vi "Stream to AVI Files (Optimized Performance) ajg.vi"() -> ()   [LabVIEW 2020]
doc: "The Stream to AVI Files (Optimized Performance) example shows how to save images to an AVI file when using a ring acquisition. This example uses a ring acquisition which is optimized for performance, but has some restrictions on the camera's image format and size. Use the Stream to AVI File example if your camera settings do not work with a ring acquisition."
uses:
  <vilib>/vision/Avi.llb/IMAQ AVI2 Codec Path.ctl
  <vilib>/vision/driver/IMAQdx.llb/IMAQdx Acquisition Mode.ctl
  <vilib>/vision/Image Controls.llb/IMAQ Image.ctl
  <vilib>/vision/driver/IMAQdx.llb/IMAQdx Buffer Number Mode.ctl
  <vilib>/Utility/High Resolution Relative Seconds.vi
  <vilib>/vision/driver/NI_Vision_Acquisition_Software.lvlib
  <resource>/objmgr/imaqdx.rc
panel:
  in  "Destination Folder":path
  in  "Skip Count":u32
  out "Images Saved Per Second":dbl
  out "Images Acquired Per Second":dbl
  in  "Images per AVI":i32=100
  out "Write Speed":dbl(graph) caption="Image File Write Speed"
  in  "Start":bool
  in  "Codec":u16(ring) items=["FF Video Codec 1 (FFV1) (NI Vision)", "Motion JPEG (NI Vision)", "VP8 (NI Vision)", "VP9 (NI Vision)", "Y800 Uncompressed Grey Scale (NI Vision)", "YUV 4:2:0 Planar (NI Vision)"]
  out "Images Behind":i32
  in  "Number of Images":i32=30
  in  "Camera Name":refnum<k21> caption="IMAQdx Session"
  in  "Stop":bool
  # "Overview: Demonstrates how to stream images to an AVI file when using a ring acquisition.\nRequirements: Vision Acquisition Software\nInstructions:\n1. Select the Camera Name\n2. Run the VI\n3. Select the Codec and click Start.\n4. Increase the Skip Count if Images Behind is greater than 0."
  # "Use the skip count to skip acquiring some images so the image logging can avoid getting behind."
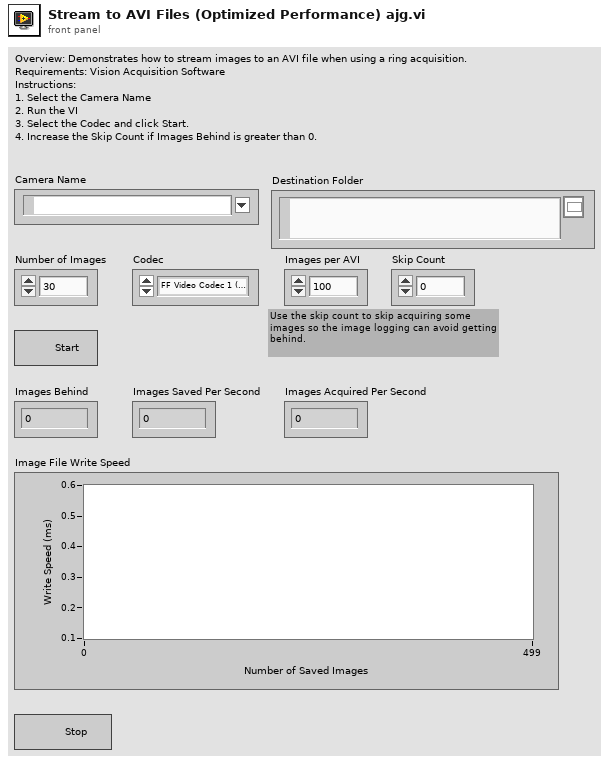
[diagram p1: front panel]
types:
  T1 = typedef "IMAQ AVI2 Codec Path.ctl" = u32
  T2 = typedef "IMAQdx.ctl" = refnum<k21>
  T3 = typedef "IMAQ Image.ctl" = refnum<image>
  T4 = typedef "NI_Vision_Acquisition_Software.lvlib/IMAQdx Acquisition Mode.ctl" = enum32{"One Shot", "Continuous"}
  T5 = typedef "NI_Vision_Acquisition_Software.lvlib/IMAQdx Buffer Number Mode.ctl" = enum32{"Next", "Last", "Buffer Number", "Every", "Last New"}
  T6 = typedef "IMAQ AVI2 Refnum.ctl" = refnum<k20>
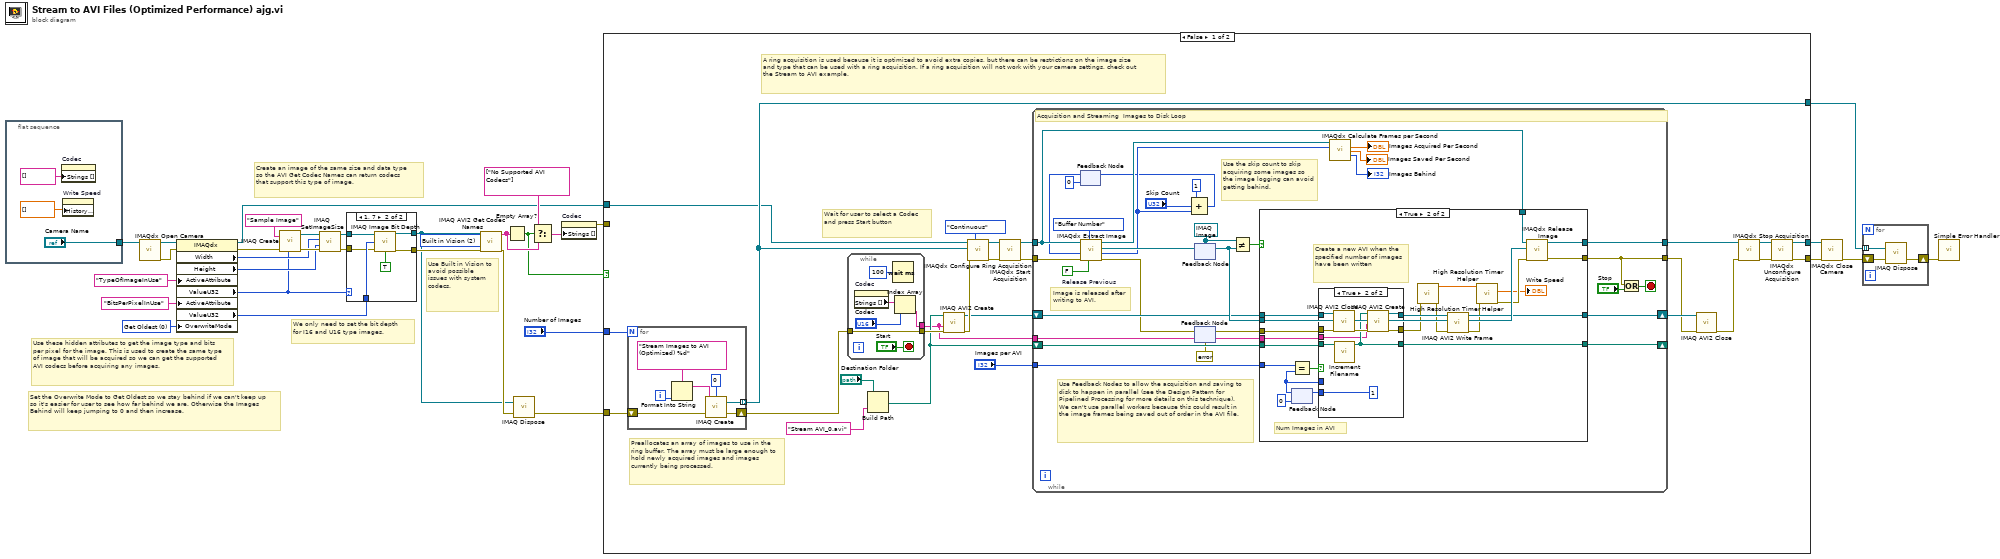
[diagram p0: block diagram]
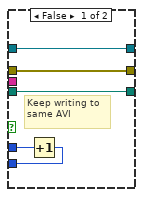
[diagram p4: hidden frame]
diagram:
  w1 = T1 2 items=["Default", "System", "Built in Vision"] ("Codec Source")
  w3 = u32 0 items=["Get Oldest"=0, "Fail"=2, "Get Newest"=3] ("OverwriteMode")
  # "Use Built in Vision to avoid possible issues with system codecs."
  # "Set the Overwrite Mode to Get Oldest so we stay behind if we can't keep up so it's easier for user to see how far behind we are. Otherwise the Images Behind will keep jumping to 0 and then increase."
  # "Create an image of the same size and data type so the AVI Get Codec Names can return codecs that support this type of image."
  # "Use these hidden attributes to get the image type and bits per pixel for the image. This is used to create the same type of image that will be acquired so we can get the supported AVI codecs before acquiring any images."
  # "We only need to set the bit depth for I16 and U16 type images."
  n1 = flat-sequence {
    tunnel: ["Camera Name"] -> w33
    frame #0 {
      n2 = property on="Codec" class="Ring (strict)"("Strings []"=string[] []) -> ()  [unwired: 2 in, 2 out]
      n3 = property on="Write Speed" class="WFChart (strict)"("History Data"=dbl[] []) -> ()  [unwired: 2 in, 2 out]
    }
  }
  n4 = call <vilib>:"IMAQdx Open Camera.vi"("Session In"=w33) -> ("error out"=w27:errorcluster, "Session Out"=w28:T2)  [unwired: 2 in, 7 out]
  n5 = property class="IMAQdx"(reference=w28, error in=w27, "ActiveAttribute"="TypeOfImageInUse", "ActiveAttribute"="BitsPerPixelInUse", "OverwriteMode"=w3) -> (reference out=w12:T2, error out=w25:errorcluster, "Width"=w21:u32, "Height"=w20:u32, "ValueU32"=w7:u32, "ValueU32"=w10:u32)
  n6 = call "IMAQ Create"("Image Name"="Sample Image", "Image Type"=w7, "error in (no error)"=w25) -> ("New Image"=w22:T3, "error out"=w23:errorcluster)  [unwired: 1 in, 1 out]
  n7 = call "IMAQ SetImageSize"("error in (no error)"=w23, "Y Resolution"=w20, "X Resolution"=w21, "Image"=w22) -> ("error out"=w9:errorcluster, "Image Out"=w8:T3)  [unwired: 1 in]
  n8 = case shown="1, 7" w7 {
    tunnel: [w37 w44] -> w13
    tunnel: w10 -> [_ w43]
    tunnel: w9 -> [w37 w42]
    tunnel: w8 -> [w38 w40]
    tunnel: [w38 w39] -> w4
    frame 0, Default {
    }
    frame 1, 7 {
      n9 = call "IMAQ Image Bit Depth"("Image"=w40, "Bit Depth (0)"=w43, "error in (no error)"=w42, "Get/Set Bit Depth? (Set)"=TRUE) -> ("Image Out"=w39:T3, "error out"=w44:errorcluster)  [unwired: 9 in, 1 out]
    }
  }
  n10 = call "IMAQ AVI2 Get Codec Names"("error in (no error)"=w13, "Codec Source"=w1, "Image"=w4) -> ("error out"=w6:errorcluster, "Codec Names"=w18:string[])  [unwired: 7 in]
  n11 = Empty Array?(array=w18) -> (empty?=w14:bool)
  n12 = call "IMAQ Dispose"("Image"=w4, "error in (no error)"=w6) -> ("error out"=w5:errorcluster)  [unwired: 4 in]
  n13 = Select(t=string[] ["No Supported AVI Codecs"], s=w14, f=w18) -> (s? t:f=w16:string[])
  n14 = property on="Codec" class="Ring (strict)"("Strings []"=w16) -> (error out=w15:errorcluster)  [unwired: 2 in, 1 out]
  n15 = case shown="False" w14 {
    tunnel: [w70 w156] -> w32
    tunnel: [w69 w157] -> w31
    tunnel: "Number of Images" -> [w63 _]
    tunnel: [w62 _] -> w29
    tunnel: w12 -> [w58 w157]
    tunnel: w5 -> [w57 w156]
    tunnel: w15 -> [_ _]
    frame False {
      # "Wait for user to select a Codec and press Start button"
      # "A ring acquisition is used because it is optimized to avoid extra copies, but there can be restrictions on the image size and type that can be used with a ring acquisition. If a ring acquisition will not work with your camera settings, check out the Stream to AVI example."
      # "Preallocates an array of images to use in the ring buffer. The array must be large enough to hold newly acquired images and images currently being processed."
      n16 = for {
        N: w63 -> [_]
        tunnel: [w154] -> w62 mode=indexing
        shift-right: [w153] -> w45
        shift-left: w57 -> [w155]
        i -> [w152]
        n17 = Format Into String(format string="Stream Images to AVI (Optimized) %d" ("Image Name"), w152) -> (resulting string=w151:string)  [unwired: 2 in, 1 out]
        n18 = call "IMAQ Create"("Border Size"=0, "Image Name"=w151, "error in (no error)"=w155) -> ("New Image"=w154:T3, "error out"=w153:errorcluster)  [unwired: 1 in, 1 out]
      }
      n19 = while {
        tunnel: w45 -> [w147]
        tunnel: [w147] -> w56
        tunnel: [w144] -> w47
        stop <- "Start" stop-if-true
        n20 = property on="Codec" class="Ring (strict)"() -> ("Strings []"=w145:string[])  [unwired: 2 in, 2 out]
        n21 = Wait (ms)(milliseconds to wait=u32 100) -> ()  [unwired: 1 out]
        n22 = Index Array(array=w145, index="Codec") -> (element=w144:string)
      }
      n23 = Build Path(base path="Destination Folder", name or relative path="Stream AVI_0.avi") -> (appended path=w48:path)
      n24 = call "IMAQ AVI2 Create"("error in (no error)"=w56, "Codec"=w47, "AVI Path"=w48) -> ("error out"=w55:errorcluster, "AVI Refnum"=w50:T6)  [unwired: 7 in]
      n25 = call <vilib>:"IMAQdx Configure Ring Acquisition.vi"("Mode"=IMAQdx_Acquisition_Mode."Continuous" ("Continuous?"), "error in"=w55, "Images"=w62, "Session In"=w58) -> ("error out"=w65:errorcluster, "Session Out"=w66:T2)  [unwired: 5 in, 1 out]
      n26 = call <vilib>:"IMAQdx Start Acquisition.vi"("error in"=w65, "Session In"=w66) -> ("error out"=w59:errorcluster, "Session Out"=w60:T2)  [unwired: 8 out]
      n27 = while {
        tunnel: w59 -> [w101]
        tunnel: w60 -> [w97]
        tunnel: [w98] -> w61
        tunnel: [w86] -> w53
        shift-right: [w99] -> w54
        shift-left: w50 -> [w85]
        tunnel: "Images per AVI" -> [w80]
        shift-right: [w81] -> _
        shift-left: w48 -> [w82]
        tunnel: w47 -> [w83]
        stop <- w88 stop-if-true
        w95 = FALSE  # Release Previous
        w91 = T3 refnum ("Image Out")
        # "Use the skip count to skip acquiring some images so the image logging can avoid getting behind."
        # "Use Feedback Nodes to allow the acquisition and saving to disk to happen in parallel (see the Design Pattern for Pipelined Processing for more details on this technique). We can't use parallel workers because this could result in the image frames being saved out of order in the AVI file."
        # "Image is released after writing to AVI."
        # "Acquisition and Streaming  Images to Disk Loop"
        n28 = feedback #1(u32 0) -> (w78:u32)
        n29 = call <vilib>:"IMAQdx Extract Image.vi"("Release Previous (true)"=w95, "Buffer Number Mode (Next)"=IMAQdx_Buffer_Number_Mode."Buffer Number" ("Buffer Number Mode"), "error in"=w101, "Buffer Number In"=w78, "Session In"=w97) -> ("error out"=w84:errorcluster, "Buffer Number Out"=w76:u32, "Image Out"=w93:T3, "Session Out"=w94:T2)  [unwired: 3 in]
        n30 = Compound Arithmetic op=ADD(u32 1 ("value"), "Skip Count", w76) -> (w73:u32)
        n31 = feedback-in #1(w73) -> ()
        n32 = feedback-in #2(w84) -> ()
        n33 = feedback #2(errorcluster {"status"=FALSE, "code"=0, "source"=""} ("error out")) -> (w92:errorcluster)
        n34 = feedback-in #3(w93) -> ()
        n35 = feedback #3(w91) -> (w89:T3)
        n36 = Not Equal?(x=w91, y=w89) -> (x != y?=w90:bool)
        n37 = case shown="True" w90 {
          tunnel: w85 -> [w103 w119]
          tunnel: w89 -> [_ w113]
          tunnel: w92 -> [w104 w118]
          tunnel: [w103 w124] -> w99
          tunnel: [w105 w127] -> w98
          tunnel: w97 -> [w105 w126]
          tunnel: [w104 w125] -> w86
          tunnel: w83 -> [_ w117]
          tunnel: w82 -> [w102 w116]
          tunnel: [w102 w114] -> w81
          tunnel: w80 -> [_ w112]
          frame False {
            # "First iteration doesn't have valid image for this pipelined stage."
          }
          frame True {
            # "Create a new AVI when the specified number of images have been written"
            # "Num Images in AVI"
            n38 = feedback #4(0) -> (w123:i32)
            n39 = Equal?(x=w112, y=w123) -> (x = y?=w120:bool)
            n40 = case shown="True" w120 {
              tunnel: [w132 1] -> w122
              tunnel: w123 -> [w133 _]
              tunnel: w119 -> [w131 w140]
              tunnel: [w131 w137] -> w115
              tunnel: w116 -> [w129 w141]
              tunnel: w118 -> [w130 w139]
              tunnel: [w130 w136] -> w111
              tunnel: [w129 w135] -> w114
              tunnel: w117 -> [_ w134]
              frame False {
                # "Keep writing to same AVI"
                n41 = Increment(x=w133) -> (x+1=w132:i32)
              }
              frame True {
                n42 = call "IMAQ AVI2 Close"("error in (no error)"=w139, "AVI Refnum"=w140) -> ("error out"=w138:errorcluster)  [unwired: 9 in]
                n43 = call "Increment Filename.vi"("Path In"=w141) -> ("Incremented Path Out"=w135:path)  [unwired: 10 in]
                n44 = call "IMAQ AVI2 Create"("error in (no error)"=w138, "Codec"=w134, "AVI Path"=w135) -> ("error out"=w136:errorcluster, "AVI Refnum"=w137:T6)  [unwired: 7 in]
              }
            }
            n45 = feedback-in #4(w122) -> ()
            n46 = call "High Resolution Timer Helper.vi"("error in (no error)"=w111) -> ("error out"=w110:errorcluster, "Current Time"=w107:dbl)  [unwired: 8 in, 1 out]
            n47 = call "IMAQ AVI2 Write Frame"("error in (no error)"=w110, "Image"=w113, "AVI Refnum"=w115) -> ("error out"=w109:errorcluster, "Image Out (duplicate)"=w128:T3, "AVI Refnum (duplicate)"=w124:T6)  [unwired: 6 in]
            n48 = call "High Resolution Timer Helper.vi"("error in (no error)"=w109, "Previous Time"=w107) -> ("error out"=w108:errorcluster, "Time Difference (ms)"=→"Write Speed":dbl)  [unwired: 7 in, 1 out]
            n49 = call <vilib>:"IMAQdx Release Image.vi"("error in"=w108, "Image"=w128, "Session In"=w126) -> ("error out"=w125:errorcluster, "Session Out"=w127:T2)  [unwired: 7 in]
          }
        }
        n50 = call <vilib>:"IMAQdx Calculate Frames per Second.vi"("Session In"=w94, "Buffer Number"=w76) -> ("Acquired Frames per Second"=→"Images Acquired Per Second":dbl, "Processed Frames per Second"=→"Images Saved Per Second":dbl, "Images Behind"=→"Images Behind":i32)  [unwired: 7 in, 4 out]
        n51 = Or(x=w86, y="Stop") -> (x .or. y?=w88:bool)
      }
      n52 = call "IMAQ AVI2 Close"("error in (no error)"=w53, "AVI Refnum"=w54) -> ("error out"=w52:errorcluster)  [unwired: 9 in]
      n53 = call <vilib>:"IMAQdx Stop Acquisition.vi"("error in"=w52, "Session In"=w61) -> ("error out"=w67:errorcluster, "Session Out"=w68:T2)  [unwired: 8 out]
      n54 = call <vilib>:"IMAQdx Unconfigure Acquisition.vi"("error in"=w67, "Session In"=w68) -> ("error out"=w70:errorcluster, "Session Out"=w69:T2)  [unwired: 8 out]
    }
    frame True {
      # "No valid AVI Codecs for the image size and image type."
    }
  }
  n55 = call <vilib>:"IMAQdx Close Camera.vi"("error in"=w32, "Session In"=w31) -> ("error out"=w19:errorcluster)  [unwired: 9 out]
  n56 = for {
    shift-right: [w159] -> w2
    shift-left: w19 -> [w160]
    tunnel: w29 -> [w158] mode=indexing
    n57 = call "IMAQ Dispose"("Image"=w158, "error in (no error)"=w160) -> ("error out"=w159:errorcluster)  [unwired: 4 in]
  }
  n58 = call <vilib>:"Simple Error Handler.vi"("error in (no error)"=w2) -> ()  [unwired: 4 in, 5 out]
